vi "Tote Steer.vi"(11 "Changed?":bool) -> (3 "f":dbl)   [LabVIEW 2014]
uses:
  Common Code/Change Detect Boolean.vi
  Robot Global Data.vi
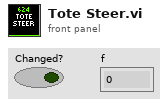
[diagram p1: front panel]
types:
  T1 = typedef "Vision Packet.ctl" = cluster{"Vision Tote":T2, "Gyro Value":dbl, "Elevator Obj Found?":bool, "Elevator Obj":T3}
  T2 = typedef "Vision Tote Data.ctl" = cluster{"Left _|":cluster{"Bounding box":cluster{"left":dbl, "top":dbl, "right":dbl, "bottom":dbl}, "Aspect Ratio":dbl, "Area Score":dbl, "X Mask":dbl, "Y Mask":dbl, "Ell":bool}, "Right |_":cluster{"Bounding box":cluster{"left":dbl, "top":dbl, "right":dbl, "bottom":dbl}, "Aspect Ratio":dbl, "Area Score":dbl, "X Mask":dbl, "Y Mask":dbl, "Ell":bool}, "Center X":dbl, "Center Y":dbl, "Angle Offset":dbl}
  T3 = typedef "Elevator Object Type.ctl" = enum16{"Grey Tote", "Yellow Tote", "Trash Can"}
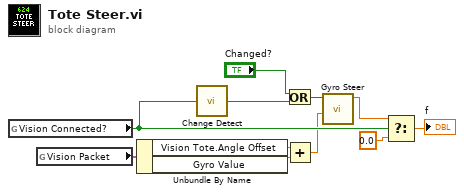
[diagram p0: block diagram]
diagram:
  n1 = global read "Robot Global Data.vi" "Vision Connected?"() -> (w11:bool)
  n2 = global read "Robot Global Data.vi" "Vision Packet"() -> (w1:T1)
  n3 = Unbundle By Name(w1) -> ("Vision Tote.Angle Offset"=w2:dbl, "Gyro Value"=w3:dbl)
  n4 = call-poly "Change Detect.vi"("In"=w11) -> ("Changed?"=w7:bool)
  n5 = Or(x="Changed?", y=w7) -> (x .or. y?=w9:bool)
  n6 = Add(x=w2, y=w3) -> (x+y=w4:dbl)
  n7 = call "Gyro Steer.vi"("Target Angle"=w4, "Changed?"=w9) -> ("X out"=w6:dbl)  [unwired: 9 in]
  n8 = Select(t=w6, s=w11, f=0.0) -> (s? t:f=→"f":dbl)
